vi "LaserPulseCalc.vi"() -> (3 "Pulse width FWHM":dbl[unit])   [LabVIEW 2023]
uses:
  <vilib>/Analysis/NI_AALPro.lvlib
panel:
  in  "Processed Data":dbl[](array[numeric])=[1020.0, 1028.0, 1026.0, 1025.0, 1027.0, 1021.0, 1030.0, 1027.0, 1030.0, 1032.0, 1031.0, 1024.0, 1026.0, 1033.0, 1028.0, 1028.0, 1029.0, 1028.0, 1039.0, 1026.0, 1037.0, 1024.0, 1033.0, 1035.0, 1029.0, 1026.0, 1031.0, 1028.0, 1033.0, 1035.0, 1042.0, 1038.0, 1035.0, 1031.0, 1035.0, 1038.0, 1045.0, 1041.0, 1043.0, 1044.0, 1036.0, 1035.0, 1032.0, 1041.0, 1042.0, 1041.0, 1033.0, 1044.0, 1039.0, 1031.0, 1036.0, 1042.0, 1042.0, 1046.0, 1037.0, 1060.0, 1039.0, 1037.0, 1036.0, 1030.0, 1038.0, 1037.0, 1045.0, 1053.0, 1048.0, 1040.0, 1049.0, 1048.0, 1034.0, 1051.0, 1045.0, 1052.0, 1051.0, 1044.0, 1045.0, 1040.0, 1047.0, 1047.0, 1053.0, 1052.0, 1052.0, 1052.0, 1051.0, 1036.0, 1044.0, 1044.0, 1056.0, 1040.0, 1050.0, 1055.0, 1052.0, 1043.0, 1051.0, 1067.0, 1053.0, 1053.0, 1064.0, 1061.0, 1056.0, 1054.0, 1061.0, 1053.0, 1056.0, 1070.0, 1075.0, 1067.0, 1075.0, 1075.0, 1062.0, 1061.0, 1068.0, 1081.0, 1088.0, 1089.0, 1078.0, 1073.0, 1076.0, 1072.0, 1080.0, 1089.0, 1094.0, 1085.0, 1081.0, 1068.0, 1066.0, 1092.0, 1074.0, 1101.0, 1090.0, 1100.0, 1087.0, 1072.0, 1089.0, 1077.0, 1089.0, 1088.0, 1087.0, 1086.0, 1094.0, 1076.0, 1074.0, 1078.0, 1078.0, 1080.0, 1091.0, 1077.0, 1079.0, 1083.0, 1079.0, 1070.0, 1087.0, 1093.0, 1083.0, 1093.0, 1086.0, 1091.0, 1084.0, 1091.0, 1095.0, 1091.0, 1090.0, 1108.0, 1106.0, 1106.0, 1100.0, 1104.0, 1101.0, 1099.0, 1118.0, 1115.0, 1124.0, 1137.0, 1126.0, 1131.0, 1118.0, 1109.0, 1114.0, 1124.0, 1149.0, 1173.0, 1152.0, 1132.0, 1120.0, 1131.0, 1125.0, 1128.0, 1159.0, 1154.0, 1139.0, 1154.0, 1140.0, 1134.0, 1130.0, 1131.0, 1152.0, 1159.0, 1160.0, 1152.0, 1138.0, 1128.0, 1122.0, 1147.0, 1147.0, 1171.0, 1152.0, 1178.0, 1165.0, 1157.0, 1146.0, 1143.0, 1148.0, 1178.0, 1186.0, 1180.0, 1165.0, 1137.0, 1132.0, 1144.0, 1148.0, 1161.0, 1170.0, 1159.0, 1166.0, 1151.0, 1159.0, 1151.0, 1156.0, 1163.0, 1182.0, 1170.0, 1200.0, 1188.0, 1186.0, 1187.0, 1186.0, 1183.0, 1207.0, 1229.0, 1229.0, 1233.0, 1217.0, 1203.0, 1176.0, 1193.0, 1213.0, 1229.0, 1253.0, 1246.0, 1236.0, 1225.0, 1217.0, 1211.0, 1225.0, 1215.0, 1257.0, 1245.0, 1231.0, 1235.0, 1218.0, 1229.0, 1225.0, 1266.0, 1296.0, 1301.0, 1310.0, 1277.0, 1251.0, 1248.0, 1271.0, 1295.0, 1313.0, 1339.0, 1323.0, 1306.0, 1273.0, 1251.0, 1234.0, 1262.0, 1299.0, 1293.0, 1293.0, 1273.0, 1255.0, 1248.0, 1241.0, 1262.0, 1267.0, 1292.0, 1312.0, 1302.0, 1313.0, 1294.0, 1307.0, 1283.0, 1293.0, 1293.0, 1321.0, 1321.0, 1338.0, 1328.0, 1346.0, 1318.0, 1331.0, 1295.0, 1333.0, 1366.0, 1376.0, 1399.0, 1364.0, 1329.0, 1314.0, 1334.0, 1354.0, 1418.0, 1463.0, 1469.0, 1460.0, 1437.0, 1393.0, 1371.0, 1400.0, 1440.0, 1534.0, 1567.0, 1517.0, 1490.0, 1447.0, 1433.0, 1444.0, 1426.0, 1511.0, 1551.0, 1558.0, 1555.0, 1483.0, 1447.0, 1445.0, 1472.0, 1528.0, 1570.0, 1559.0, 1547.0, 1523.0, 1475.0, 1469.0, 1517.0, 1535.0, 1566.0, 1567.0, 1563.0, 1545.0, 1531.0, 1518.0, 1530.0, 1544.0, 1571.0, 1626.0, 1607.0, 1580.0, 1564.0, 1537.0, 1519.0, 1527.0, 1580.0, 1614.0, 1628.0, 1666.0, 1660.0, 1589.0, 1590.0, 1587.0, 1582.0, 1667.0, 1707.0, 1768.0, 1781.0, 1735.0, 1730.0, 1652.0, 1659.0, 1678.0, 1739.0, 1854.0, 1875.0, 1864.0, 1854.0, 1779.0, 1749.0, 1748.0, 1828.0, 1824.0, 1915.0, 1939.0, 1876.0, 1812.0, 1775.0, 1732.0, 1730.0, 1841.0, 1977.0, 1969.0, 2000.0, 1916.0, 1872.0, 1786.0, 1813.0, 1859.0, 2022.0, 2098.0, 2143.0, 2052.0, 1921.0, 1857.0, 1824.0, 1853.0, 1926.0, 1963.0, 2008.0, 1949.0, 1882.0, 1784.0, 1764.0, 1774.0, 1803.0, 1877.0, 1890.0, 1861.0, 1812.0, 1757.0, 1763.0, 1762.0, 1739.0, 1797.0, 1824.0, 1901.0, 1863.0, 1824.0, 1781.0, 1761.0, 1702.0, 1725.0, 1774.0, 1846.0, 1860.0, 1883.0, 1867.0, 1815.0, 1842.0, 1767.0, 1808.0, 1914.0, 1963.0, 2024.0, 1992.0, 1920.0, 1829.0, 1802.0, 1820.0, 1895.0, 1921.0, 2042.0, 2057.0, 2034.0, 1986.0, 1908.0, 1861.0, 1854.0, 1932.0, 2094.0, 2199.0, 2223.0, 2124.0, 2051.0, 1945.0, 1923.0, 2011.0, 2121.0, 2184.0, 2197.0, 2150.0, 2046.0, 1891.0, 1866.0, 1842.0, 1919.0, 1995.0, 2093.0, 2096.0, 2035.0, 1959.0, 1881.0, 1866.0, 1877.0, 1965.0, 2072.0, 2041.0, 2108.0, 2041.0, 1959.0, 1924.0, 1908.0, 1925.0, 1932.0, 1988.0, 2010.0, 2043.0, 1965.0, 1888.0, 1920.0, 1934.0, 1983.0, 2063.0, 2077.0, 2078.0, 2032.0, 1967.0, 1914.0, 1945.0, 1912.0, 1969.0, 2000.0, 2120.0, 2151.0, 2173.0, 2118.0, 2077.0, 1975.0, 2015.0, 2081.0, 2181.0, 2314.0, 2284.0, 2225.0, 2119.0, 2031.0, 1980.0, 2070.0, 2174.0, 2297.0, 2316.0, 2339.0, 2183.0, 2096.0, 1936.0, 1952.0, 2066.0, 2124.0, 2226.0, 2292.0, 2180.0, 2072.0, 2042.0, 2059.0, 2046.0, 2129.0, 2226.0, 2320.0, 2328.0, 2196.0, 2066.0, 1990.0, 1958.0, 2016.0, 2130.0, 2241.0, 2292.0, 2245.0, 2096.0, 2008.0, 1982.0, 1995.0, 2078.0, 2155.0, 2109.0, 2128.0, 2061.0, 2036.0, 1981.0, 1977.0, 1919.0, 2006.0, 2061.0, 2069.0, 2118.0, 2071.0, 2131.0, 2069.0, 2027.0, 2081.0, 2056.0, 2153.0, 2156.0, 2168.0, 2153.0, 2162.0, 2138.0, 2114.0, 2137.0, 2214.0, 2226.0, 2302.0, 2304.0, 2256.0, 2225.0, 2133.0, 2129.0, 2131.0, 2156.0, 2294.0, 2299.0, 2270.0, 2305.0, 2271.0, 2176.0, 2178.0, 2211.0, 2287.0, 2411.0, 2427.0, 2387.0, 2267.0, 2156.0, 2090.0, 2160.0, 2218.0, 2327.0, 2443.0, 2337.0, 2215.0, 2079.0, 1983.0, 2004.0, 2082.0, 2157.0, 2250.0, 2231.0, 2134.0, 2076.0, 2002.0, 1914.0, 1915.0, 1968.0, 2053.0, 2132.0, 2203.0, 2139.0, 2105.0, 2032.0, 1974.0, 1915.0, 1985.0, 2052.0, 2081.0, 2063.0, 2125.0, 2032.0, 1965.0, 1923.0, 1928.0, 1968.0, 2013.0, 2016.0, 2062.0, 2070.0, 1995.0, 1962.0, 1896.0, 1988.0, 1989.0, 2003.0, 2138.0, 2135.0, 2146.0, 2128.0, 2124.0, 1991.0, 1995.0, 2005.0, 2068.0, 2190.0, 2253.0, 2182.0, 2128.0, 2005.0, 1994.0, 1993.0, 2080.0, 2140.0, 2142.0, 2161.0, 2111.0, 2017.0, 1961.0, 1944.0, 2034.0, 2085.0, 2146.0, 2162.0, 2159.0, 2101.0, 1980.0, 1894.0, 1821.0, 1875.0, 1941.0, 2020.0, 2111.0, 2069.0, 1986.0, 1905.0, 1825.0, 1769.0, 1812.0, 1949.0, 2012.0, 2031.0, 2010.0, 1878.0, 1833.0, 1758.0, 1766.0, 1798.0, 1816.0, 1839.0, 1826.0, 1769.0, 1719.0, 1706.0, 1705.0, 1684.0, 1682.0, 1689.0, 1747.0, 1728.0, 1714.0, 1668.0, 1692.0, 1654.0, 1657.0, 1695.0, 1718.0, 1750.0, 1800.0, 1773.0, 1732.0, 1699.0, 1663.0, 1665.0, 1647.0, 1708.0, 1764.0, 1755.0, 1727.0, 1710.0, 1667.0, 1615.0, 1616.0, 1645.0, 1696.0, 1766.0, 1753.0, 1725.0, 1649.0, 1638.0, 1591.0, 1555.0, 1634.0, 1704.0, 1745.0, 1794.0, 1774.0, 1731.0, 1662.0, 1599.0, 1631.0, 1669.0, 1734.0, 1759.0, 1781.0, 1738.0, 1636.0, 1627.0, 1597.0, 1586.0, 1581.0, 1603.0, 1599.0, 1597.0, 1545.0, 1518.0, 1467.0, 1470.0, 1461.0, 1472.0, 1515.0, 1515.0, 1534.0, 1516.0, 1460.0, 1450.0, 1448.0, 1433.0, 1464.0, 1504.0, 1478.0, 1469.0, 1489.0, 1451.0, 1440.0, 1429.0, 1437.0, 1434.0, 1472.0, 1491.0, 1482.0, 1429.0, 1426.0, 1412.0, 1389.0, 1374.0, 1399.0, 1405.0, 1431.0, 1411.0, 1432.0, 1402.0, 1404.0, 1370.0, 1378.0, 1344.0, 1351.0, 1409.0, 1424.0, 1396.0, 1429.0, 1409.0, 1394.0, 1372.0, 1412.0, 1418.0, 1463.0, 1456.0, 1451.0, 1425.0, 1353.0, 1340.0, 1339.0, 1413.0, 1458.0, 1442.0, 1427.0, 1409.0, 1355.0, 1311.0, 1294.0, 1319.0, 1345.0, 1398.0, 1394.0, 1402.0, 1381.0, 1332.0, 1311.0, 1319.0, 1315.0, 1345.0, 1365.0, 1375.0, 1371.0, 1357.0, 1314.0, 1290.0, 1306.0, 1305.0, 1316.0, 1357.0, 1351.0, 1328.0, 1323.0, 1290.0, 1275.0, 1288.0, 1270.0, 1279.0, 1276.0, 1292.0, 1285.0, 1287.0, 1267.0, 1267.0, 1277.0, 1251.0, 1257.0, 1294.0, 1291.0, 1324.0, 1288.0, 1303.0, 1292.0, 1264.0, 1257.0, 1277.0, 1270.0, 1275.0, 1284.0, 1278.0, 1274.0, 1247.0, 1251.0, 1241.0, 1272.0, 1270.0, 1271.0, 1292.0, 1279.0, 1254.0, 1251.0, 1240.0, 1228.0, 1239.0, 1292.0, 1289.0, 1310.0, 1297.0, 1268.0, 1260.0, 1238.0, 1230.0, 1246.0, 1272.0, 1303.0, 1291.0, 1281.0, 1258.0, 1224.0, 1185.0, 1174.0, 1189.0, 1202.0, 1239.0, 1244.0, 1216.0, 1219.0, 1177.0, 1184.0, 1166.0, 1182.0, 1184.0, 1211.0, 1191.0, 1189.0, 1165.0, 1164.0, 1171.0, 1155.0, 1164.0, 1156.0, 1193.0, 1180.0, 1175.0, 1184.0, 1156.0, 1164.0, 1142.0, 1142.0, 1152.0, 1156.0, 1160.0, 1154.0, 1183.0, 1156.0, 1146.0, 1138.0, 1142.0, 1126.0, 1145.0, 1143.0, 1175.0, 1151.0, 1154.0, 1151.0, 1157.0, 1123.0, 1136.0, 1148.0, 1164.0, 1184.0, 1173.0, 1171.0, 1143.0, 1137.0, 1128.0, 1124.0, 1124.0, 1163.0, 1165.0, 1148.0, 1143.0, 1131.0, 1128.0, 1111.0, 1124.0, 1124.0, 1127.0, 1131.0, 1129.0, 1118.0, 1103.0, 1109.0, 1098.0, 1100.0, 1112.0, 1134.0, 1105.0, 1118.0, 1120.0, 1108.0, 1104.0, 1110.0, 1094.0, 1105.0, 1109.0, 1114.0, 1135.0]
  in  "Multi-Acquisitions.Array of Wavelengths":dbl[](array[numeric])=[833.656, 833.688, 833.72, 833.753, 833.785, 833.817, 833.85, 833.882, 833.915, 833.947, 833.979, 834.012, 834.044, 834.076, 834.109, 834.141, 834.173, 834.206, 834.238, 834.27, 834.303, 834.335, 834.367, 834.4, 834.432, 834.464, 834.497, 834.529, 834.561, 834.594, 834.626, 834.658, 834.691, 834.723, 834.755, 834.788, 834.82, 834.852, 834.885, 834.917, 834.949, 834.981, 835.014, 835.046, 835.078, 835.111, 835.143, 835.175, 835.208, 835.24, 835.272, 835.304, 835.337, 835.369, 835.401, 835.434, 835.466, 835.498, 835.53, 835.563, 835.595, 835.627, 835.659, 835.692, 835.724, 835.756, 835.788, 835.821, 835.853, 835.885, 835.917, 835.95, 835.982, 836.014, 836.046, 836.079, 836.111, 836.143, 836.175, 836.208, 836.24, 836.272, 836.304, 836.337, 836.369, 836.401, 836.433, 836.466, 836.498, 836.53, 836.562, 836.594, 836.627, 836.659, 836.691, 836.723, 836.755, 836.788, 836.82, 836.852, 836.884, 836.916, 836.949, 836.981, 837.013, 837.045, 837.077, 837.11, 837.142, 837.174, 837.206, 837.238, 837.271, 837.303, 837.335, 837.367, 837.399, 837.431, 837.464, 837.496, 837.528, 837.56, 837.592, 837.624, 837.657, 837.689, 837.721, 837.753, 837.785, 837.817, 837.849, 837.882, 837.914, 837.946, 837.978, 838.01, 838.042, 838.074, 838.107, 838.139, 838.171, 838.203, 838.235, 838.267, 838.299, 838.331, 838.364, 838.396, 838.428, 838.46, 838.492, 838.524, 838.556, 838.588, 838.621, 838.653, 838.685, 838.717, 838.749, 838.781, 838.813, 838.845, 838.877, 838.909, 838.941, 838.974, 839.006, 839.038, 839.07, 839.102, 839.134, 839.166, 839.198, 839.23, 839.262, 839.294, 839.326, 839.358, 839.391, 839.423, 839.455, 839.487, 839.519, 839.551, 839.583, 839.615, 839.647, 839.679, 839.711, 839.743, 839.775, 839.807, 839.839, 839.871, 839.903, 839.935, 839.967, 839.999, 840.031, 840.063, 840.095, 840.127, 840.16, 840.192, 840.224, 840.256, 840.288, 840.32, 840.352, 840.384, 840.416, 840.448, 840.48, 840.512, 840.544, 840.576, 840.608, 840.64, 840.672, 840.704, 840.736, 840.768, 840.8, 840.832, 840.864, 840.896, 840.927, 840.959, 840.991, 841.023, 841.055, 841.087, 841.119, 841.151, 841.183, 841.215, 841.247, 841.279, 841.311, 841.343, 841.375, 841.407, 841.439, 841.471, 841.503, 841.535, 841.567, 841.599, 841.631, 841.662, 841.694, 841.726, 841.758, 841.79, 841.822, 841.854, 841.886, 841.918, 841.95, 841.982, 842.014, 842.046, 842.078, 842.109, 842.141, 842.173, 842.205, 842.237, 842.269, 842.301, 842.333, 842.365, 842.397, 842.428, 842.46, 842.492, 842.524, 842.556, 842.588, 842.62, 842.652, 842.684, 842.715, 842.747, 842.779, 842.811, 842.843, 842.875, 842.907, 842.939, 842.97, 843.002, 843.034, 843.066, 843.098, 843.13, 843.162, 843.193, 843.225, 843.257, 843.289, 843.321, 843.353, 843.385, 843.416, 843.448, 843.48, 843.512, 843.544, 843.576, 843.607, 843.639, 843.671, 843.703, 843.735, 843.766, 843.798, 843.83, 843.862, 843.894, 843.926, 843.957, 843.989, 844.021, 844.053, 844.085, 844.116, 844.148, 844.18, 844.212, 844.244, 844.275, 844.307, 844.339, 844.371, 844.403, 844.434, 844.466, 844.498, 844.53, 844.561, 844.593, 844.625, 844.657, 844.688, 844.72, 844.752, 844.784, 844.816, 844.847, 844.879, 844.911, 844.943, 844.974, 845.006, 845.038, 845.07, 845.101, 845.133, 845.165, 845.197, 845.228, 845.26, 845.292, 845.323, 845.355, 845.387, 845.419, 845.45, 845.482, 845.514, 845.546, 845.577, 845.609, 845.641, 845.672, 845.704, 845.736, 845.768, 845.799, 845.831, 845.863, 845.894, 845.926, 845.958, 845.989, 846.021, 846.053, 846.085, 846.116, 846.148, 846.18, 846.211, 846.243, 846.275, 846.306, 846.338, 846.37, 846.401, 846.433, 846.465, 846.496, 846.528, 846.56, 846.591, 846.623, 846.655, 846.686, 846.718, 846.75, 846.781, 846.813, 846.845, 846.876, 846.908, 846.94, 846.971, 847.003, 847.034, 847.066, 847.098, 847.129, 847.161, 847.193, 847.224, 847.256, 847.287, 847.319, 847.351, 847.382, 847.414, 847.446, 847.477, 847.509, 847.54, 847.572, 847.604, 847.635, 847.667, 847.698, 847.73, 847.762, 847.793, 847.825, 847.856, 847.888, 847.92, 847.951, 847.983, 848.014, 848.046, 848.077, 848.109, 848.141, 848.172, 848.204, 848.235, 848.267, 848.298, 848.33, 848.362, 848.393, 848.425, 848.456, 848.488, 848.519, 848.551, 848.582, 848.614, 848.645, 848.677, 848.709, 848.74, 848.772, 848.803, 848.835, 848.866, 848.898, 848.929, 848.961, 848.992, 849.024, 849.055, 849.087, 849.118, 849.15, 849.181, 849.213, 849.244, 849.276, 849.308, 849.339, 849.371, 849.402, 849.434, 849.465, 849.497, 849.528, 849.559, 849.591, 849.622, 849.654, 849.685, 849.717, 849.748, 849.78, 849.811, 849.843, 849.874, 849.906, 849.937, 849.969, 850.0, 850.032, 850.063, 850.095, 850.126, 850.158, 850.189, 850.22, 850.252, 850.283, 850.315, 850.346, 850.378, 850.409, 850.441, 850.472, 850.503, 850.535, 850.566, 850.598, 850.629, 850.661, 850.692, 850.723, 850.755, 850.786, 850.818, 850.849, 850.881, 850.912, 850.943, 850.975, 851.006, 851.038, 851.069, 851.1, 851.132, 851.163, 851.195, 851.226, 851.257, 851.289, 851.32, 851.352, 851.383, 851.414, 851.446, 851.477, 851.508, 851.54, 851.571, 851.603, 851.634, 851.665, 851.697, 851.728, 851.759, 851.791, 851.822, 851.854, 851.885, 851.916, 851.948, 851.979, 852.01, 852.042, 852.073, 852.104, 852.136, 852.167, 852.198, 852.23, 852.261, 852.292, 852.324, 852.355, 852.386, 852.418, 852.449, 852.48, 852.512, 852.543, 852.574, 852.606, 852.637, 852.668, 852.7, 852.731, 852.762, 852.794, 852.825, 852.856, 852.887, 852.919, 852.95, 852.981, 853.013, 853.044, 853.075, 853.106, 853.138, 853.169, 853.2, 853.232, 853.263, 853.294, 853.325, 853.357, 853.388, 853.419, 853.451, 853.482, 853.513, 853.544, 853.576, 853.607, 853.638, 853.669, 853.701, 853.732, 853.763, 853.794, 853.826, 853.857, 853.888, 853.919, 853.951, 853.982, 854.013, 854.044, 854.075, 854.107, 854.138, 854.169, 854.2, 854.232, 854.263, 854.294, 854.325, 854.356, 854.388, 854.419, 854.45, 854.481, 854.513, 854.544, 854.575, 854.606, 854.637, 854.669, 854.7, 854.731, 854.762, 854.793, 854.824, 854.856, 854.887, 854.918, 854.949, 854.98, 855.012, 855.043, 855.074, 855.105, 855.136, 855.167, 855.199, 855.23, 855.261, 855.292, 855.323, 855.354, 855.386, 855.417, 855.448, 855.479, 855.51, 855.541, 855.572, 855.604, 855.635, 855.666, 855.697, 855.728, 855.759, 855.79, 855.822, 855.853, 855.884, 855.915, 855.946, 855.977, 856.008, 856.039, 856.07, 856.102, 856.133, 856.164, 856.195, 856.226, 856.257, 856.288, 856.319, 856.35, 856.382, 856.413, 856.444, 856.475, 856.506, 856.537, 856.568, 856.599, 856.63, 856.661, 856.692, 856.723, 856.755, 856.786, 856.817, 856.848, 856.879, 856.91, 856.941, 856.972, 857.003, 857.034, 857.065, 857.096, 857.127, 857.158, 857.189, 857.22, 857.251, 857.283, 857.314, 857.345, 857.376, 857.407, 857.438, 857.469, 857.5, 857.531, 857.562, 857.593, 857.624, 857.655, 857.686, 857.717, 857.748, 857.779, 857.81, 857.841, 857.872, 857.903, 857.934, 857.965, 857.996, 858.027, 858.058, 858.089, 858.12, 858.151, 858.182, 858.213, 858.244, 858.275, 858.306, 858.337, 858.368, 858.399, 858.43, 858.461, 858.492, 858.523, 858.554, 858.585, 858.616, 858.647, 858.678, 858.709, 858.739, 858.77, 858.801, 858.832, 858.863, 858.894, 858.925, 858.956, 858.987, 859.018, 859.049, 859.08, 859.111, 859.142, 859.173, 859.204, 859.235, 859.265, 859.296, 859.327, 859.358, 859.389, 859.42, 859.451, 859.482, 859.513, 859.544, 859.575, 859.606, 859.636, 859.667, 859.698, 859.729, 859.76, 859.791, 859.822, 859.853, 859.884, 859.914, 859.945, 859.976, 860.007, 860.038, 860.069, 860.1, 860.131, 860.162, 860.192, 860.223, 860.254, 860.285, 860.316, 860.347, 860.378, 860.408, 860.439, 860.47, 860.501, 860.532, 860.563, 860.594, 860.624, 860.655, 860.686, 860.717, 860.748, 860.779, 860.809, 860.84, 860.871, 860.902, 860.933, 860.964, 860.994, 861.025, 861.056, 861.087, 861.118, 861.148, 861.179, 861.21, 861.241, 861.272, 861.302, 861.333, 861.364, 861.395, 861.426, 861.456, 861.487, 861.518, 861.549, 861.58, 861.61, 861.641, 861.672, 861.703, 861.734, 861.764, 861.795, 861.826, 861.857, 861.887, 861.918, 861.949, 861.98, 862.01, 862.041, 862.072, 862.103, 862.133, 862.164, 862.195, 862.226, 862.256, 862.287, 862.318, 862.349, 862.379, 862.41, 862.441, 862.472, 862.502, 862.533, 862.564, 862.595, 862.625, 862.656, 862.687, 862.717, 862.748, 862.779, 862.81, 862.84, 862.871, 862.902, 862.932, 862.963, 862.994, 863.025, 863.055, 863.086, 863.117, 863.147, 863.178, 863.209, 863.239, 863.27, 863.301, 863.331, 863.362, 863.393, 863.423, 863.454, 863.485, 863.515, 863.546, 863.577, 863.607, 863.638, 863.669, 863.699, 863.73, 863.761, 863.791, 863.822, 863.853, 863.883, 863.914, 863.945, 863.975, 864.006, 864.037, 864.067, 864.098, 864.129, 864.159, 864.19, 864.22, 864.251, 864.282, 864.312, 864.343, 864.374, 864.404, 864.435, 864.465, 864.496, 864.527, 864.557, 864.588, 864.618, 864.649, 864.68, 864.71, 864.741, 864.771, 864.802, 864.833, 864.863, 864.894, 864.924, 864.955, 864.985, 865.016, 865.047, 865.077, 865.108, 865.138, 865.169, 865.2, 865.23, 865.261, 865.291, 865.322, 865.352, 865.383, 865.413, 865.444, 865.475, 865.505, 865.536, 865.566, 865.597, 865.627, 865.658, 865.688, 865.719, 865.749, 865.78, 865.81, 865.841]
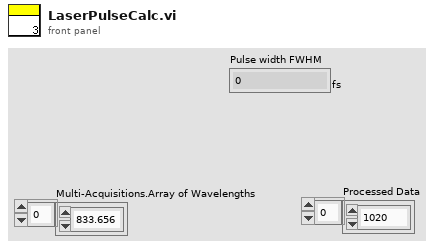
[diagram p1: front panel]
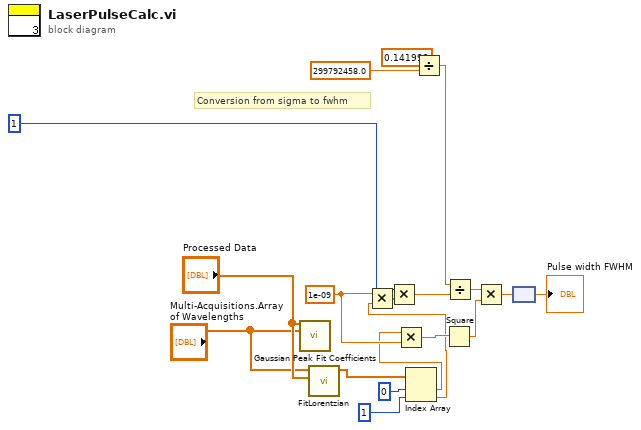
[diagram p0: block diagram]
diagram:
  w8 = 1e-09 ("x")
  # "Conversion from sigma to fwhm"
  n1 = call <vilib>:"Gaussian Peak Fit Coefficients.vi"("Y"="Processed Data", "X"="Multi-Acquisitions.Array of Wavelengths") -> ()  [unwired: 10 in, 4 out]
  n2 = call "FitLorentzian.vi"("y"="Processed Data", "x"="Multi-Acquisitions.Array of Wavelengths") -> ("best fit parameters"=w7:dbl[])  [unwired: 9 in]
  n3 = Index Array(array=w7, index #1=0 ("index"), index #2=1 ("index")) -> (element #1=w3:dbl, element #2=w4:dbl)
  n4 = Multiply(x=w8, y=w4) -> (x*y=w9:dbl)
  n5 = Multiply(x=1 ("Numeric"), y=w9) -> (x*y=w15:dbl)
  n6 = Multiply(x=w3, y=w8) -> (x*y=w10:dbl)
  n7 = Divide(x=0.141999 ("Numeric"), y=299792458.0 ("Numeric")) -> (x/y=w16:dbl)
  n8 = Square(x=w10) -> (x^2=w14:dbl)
  n9 = Divide(x=w16, y=w15) -> (x/y=w13:dbl)
  n10 = Multiply(x=w13, y=w14) -> (x*y=w12:dbl)
  n11 = node(w12) -> (→"Pulse width FWHM":dbl[unit])
